vi "Multiply Quaternions.vi"   [LabVIEW 2017, in "NI_Kinematics.lvlib"]
doc: "Returns the <B>product</B> of two quaternions or a quaternion and a scalar number. Wire data to the <B>y</B> input to determine the polymorphic instance to use or manually select the instance."
uses:
  <vilib>/robotics/Kinematics/NI_Kinematics.lvlib
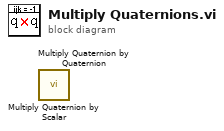
[diagram p0: block diagram]
diagram:
  n1 = call <vilib>:"Multiply Quaternion by Scalar.vi"() -> ()  [unwired: 2 in, 1 out]
  n2 = call <vilib>:"Multiply Quaternion by Quaternion.vi"() -> ()  [unwired: 2 in, 1 out]
